vi "Custom-error-definitions.vi"(8 "error in (no error)":errorcluster, 11 "Language":T1) -> (0 "error out":errorcluster, 4 "Descriptions":string[](array[string])=["AccessDenied: TCP/IP networking access was denied.", "Communications: TCP/IP network communications error occured.", "NotConnected: Client is not connected to the server.", "IllegalClientId: Internal error.", "InvalidPersistState: Internal error.", "ServerNameNotFound: Requested server name is not valid.", "InvalidParameter: Bad parameter to a method call.", "Network: TCP/IP networking error.", "DataNotFound: Requested data file not found.", "PathNotFound: Specified path does not exist.", "Access: Access to server file system was denied.", "LocalAccess: Access to the client file system was denied or Server is under control of a local pendant.", "DataUnknown: XML data type is unknown.", "EventHandling: Internal event processing error.", "NotAvailable: Server is not currently available.", "Aborting: Server is currently aborting.", "Aborted: Server action was aborted.", "Exception: Internal error.", "Timeout: Requested action timed out.", "NoData: Thre requested fixed data was empty.", "DataExists: Destination file already exists and over-write not specified.", "RemoteAccess: Server is already connected to a client.", "StateError: Server is in error state and unavailable.", "BufferFull: Streaming data transmit buffer is full."], 6 "Error codes":i32[](array[numeric]))   [LabVIEW 2013, in "CameraVision.lvlib" / "CV-Client.lvclass"]
doc: "This function contains a table which provides the relation between an error code and the error description (text).\nThe error range can be modified through the error code offset. The codes should correspond to those used by the 'Invoke-error' function.\nOptionally supports multiple languages."
uses:
  CV-Client.lvclass
  Errors/Languages.ctl
  Errors/CV-Errors.lvclass
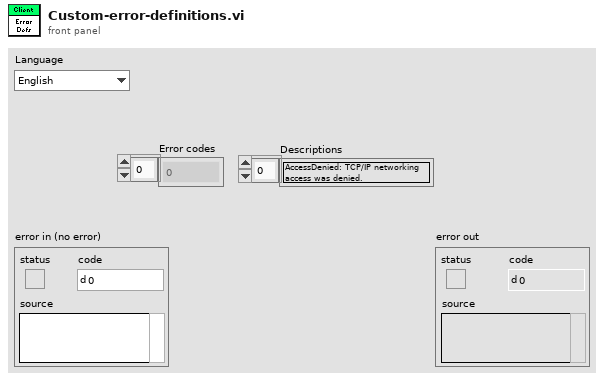
[diagram p1: front panel]
types:
  T1 = typedef "CameraVision.lvlib/CV-Errors.lvclass/Languages.ctl" = enum16{"English"}
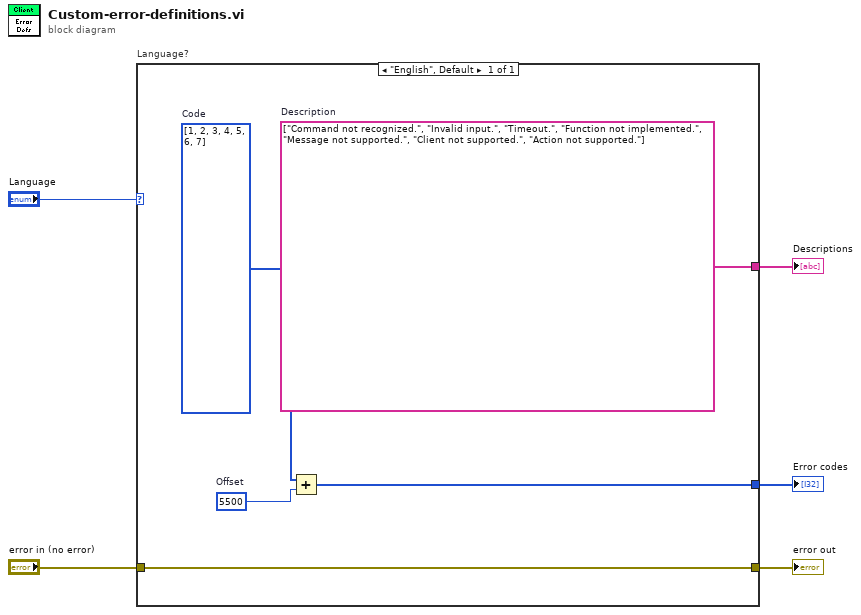
[diagram p0: block diagram]
diagram:
  n1 = case "Language?" shown="\"English\", Default" "Language" {
    tunnel: [w8] -> w5
    tunnel: [w7] -> w4
    tunnel: "error in (no error)" -> [w6]
    tunnel: [w6] -> w1
    frame "English", Default {
      w10 = 5500  # Offset
      w9 = i32[] [1, 2, 3, 4, 5, 6, 7]  # Code
      w8 = string[] ["Command not recognized.", "Invalid input.", "Timeout.", "Function not implemented.", "Message not supported.", "Client not supported.", "Action not supported."]  # Description
      n2 = Add(x=w9, y=w10) -> (x+y=w7:i32[])
    }
  }
  "Descriptions" <- w5
  "Error codes" <- w4
  "error out" <- w1
